vi "Excel_Set_Orientation.vi"(0 "Excel._Worksheet":refnum<k7>, 7 "orientation (portrait)":u16, 11 "error in (no error)":errorcluster) -> (15 "error out":errorcluster)   [LabVIEW 2010, in "NI_ReportGenerationToolkit.lvlib"]
uses:
  <vilib>/addons/_office/NI_ReportGenerationToolkit.lvlib
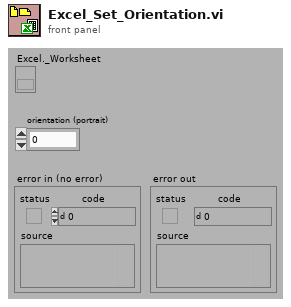
[diagram p1: front panel]
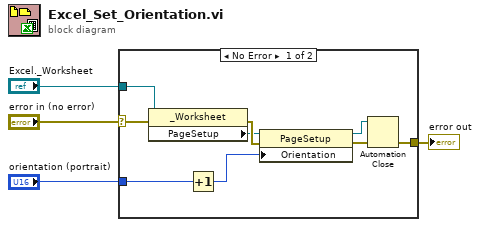
[diagram p0: block diagram]
diagram:
  n1 = case shown="No Error" "error in (no error)" {
    selector: "error in (no error)" -> [w5 w14]
    tunnel: "orientation (portrait)" -> [w12 _]
    tunnel: [w11 w14] -> w3
    tunnel: "Excel._Worksheet" -> [w9 _]
    frame No Error {
      n2 = property class="_Worksheet"(reference=w9, error in=w5) -> (error out=w10:errorcluster, "PageSetup"=w6:refnum<k7>)  [unwired: 1 out]
      n3 = Increment(x=w12) -> (x+1=w13:u16)
      n4 = property class="PageSetup"(reference=w6, error in=w10, "Orientation"=w13) -> (reference out=w8:refnum<k7>, error out=w7:errorcluster)
      n5 = Automation Close(3:w7, 5:w8) -> (0:w11:errorcluster)
    }
    frame Error {
    }
  }
  "error out" <- w3
